vi "Notify.vi"(8 "error in (no error)":errorcluster, 9 "ICallResult":refnum<class "ICallResult.lvclass">, 10 "Events":refnum<class "Events.lvclass">, 11 "ICallRequest in":refnum<class "ICallRequest.lvclass">) -> (0 "error out":errorcluster, 3 "ICallRequest out":refnum<class "ICallRequest.lvclass">)   [LabVIEW 2020, in "wamplv.lvlib" / "ICallRequest.lvclass"]
uses:
  ICallRequest.lvclass
  ICallResult/ICallResult.lvclass
  Events/EventsParent/Events.lvclass
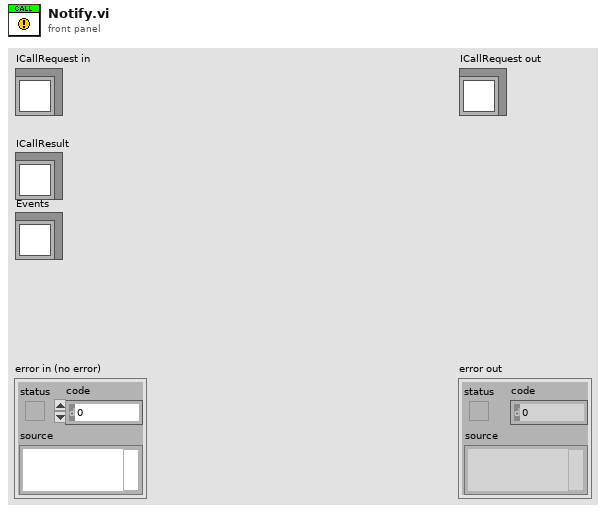
[diagram p1: front panel]
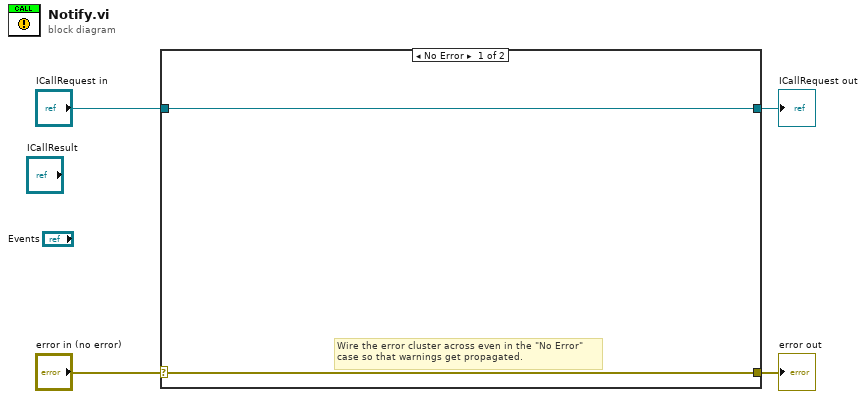
[diagram p0: block diagram]
diagram:
  n1 = case shown="No Error" "error in (no error)" {
    selector: "error in (no error)" -> [w5 w8]
    tunnel: [w5 w8] -> w3
    tunnel: [w6 w7] -> w1
    tunnel: "ICallRequest in" -> [w6 w7]
    frame No Error {
      # "Wire the error cluster across even in the \"No Error\"\ncase so that warnings get propagated."
    }
    frame Error {
    }
  }
  "error out" <- w3
  "ICallRequest out" <- w1
